vi "to_SGL.vi"(8 "error_in":errorcluster, 10 "variable_start_index":i32, 11 "byte_array":u8[](array[numeric])) -> (0 "error_out":errorcluster, 3 "SGL":sgl)   [LabVIEW 2020]
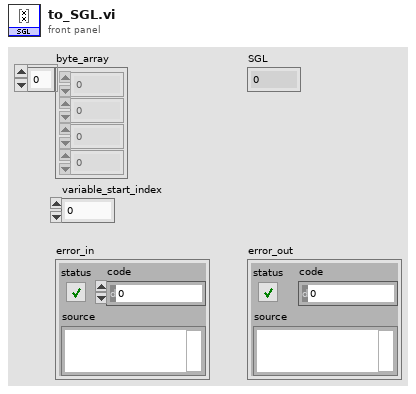
[diagram p1: front panel]
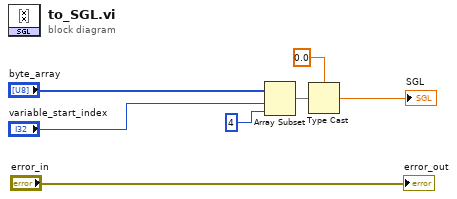
[diagram p0: block diagram]
diagram:
  n1 = Array Subset(array="byte_array", index="variable_start_index", length=4) -> (w3:u8[])
  n2 = Type Cast(type=sgl 0.0 ("SGL"), x=w3) -> (*(type *) &x=→"SGL":sgl)
  "error_out" <- "error_in"
